vi "LabviewEnvironment.vi"() -> ()   [LabVIEW 2019]
uses:
  <vilib>/Waveform/DWDTOps.llb/DWDT Analog to Digital.vi
  <vilib>/measure/NI_MABase.lvlib
panel:
  out "Digital Waveform Graph":digitalwaveform(graph)
  in  "phase":dbl format="%.2p"
  in  "amplitude":dbl=1.0 format="%0.2p"
  in  "frequency":dbl=10.0 format="%0.2p"
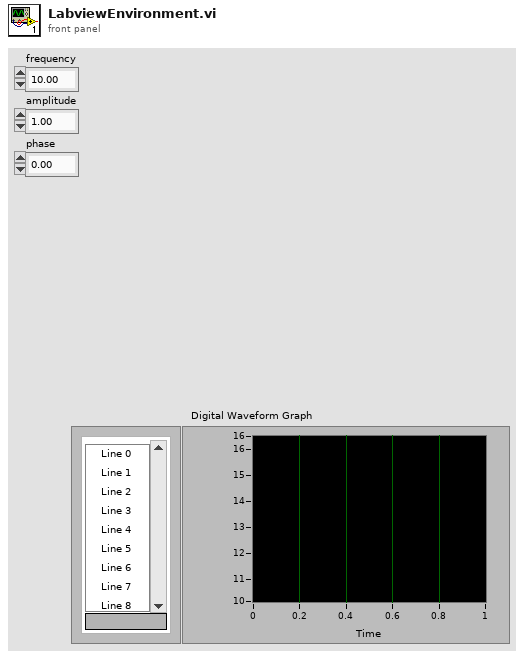
[diagram p1: front panel]
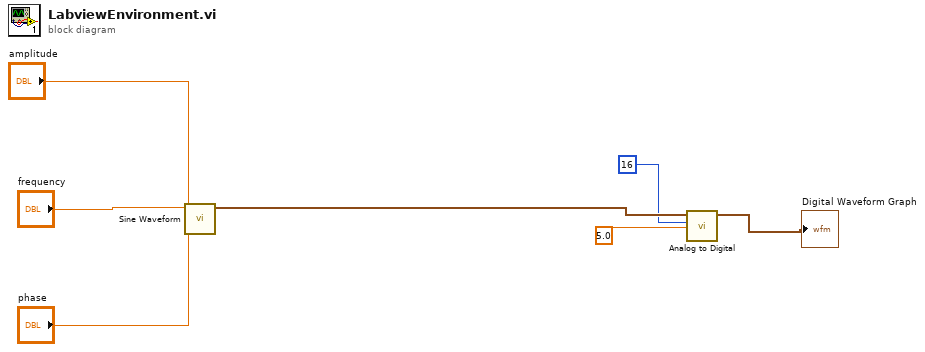
[diagram p0: block diagram]
diagram:
  n1 = call <vilib>:"Sine Waveform.vi"("phase"="phase", "amplitude"="amplitude", "frequency"="frequency") -> ("signal out"=w4:waveform(dbl))  [unwired: 7 in, 1 out]
  n2 = call-poly <vilib>:"Analog to Digital.vi"("full-scale range (pk-pk)"=5.0, "resolution (16 bit)"=16, "analog waveform"=w4) -> ("digital waveform"=→"Digital Waveform Graph":digitalwaveform)  [unwired: 5 in, 3 out]
